vi "tutorialE11.vi"() -> ()   [LabVIEW 2017]
uses:
  Control 1.ctl
panel:
  in  "Delay (ms)":u32
  out "Count":dbl
  in  "# of Iterations":T1 scale=0.0..100.0
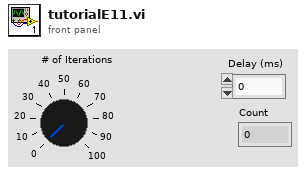
[diagram p1: front panel]
types:
  T1 = typedef "Control 1.ctl" = dbl
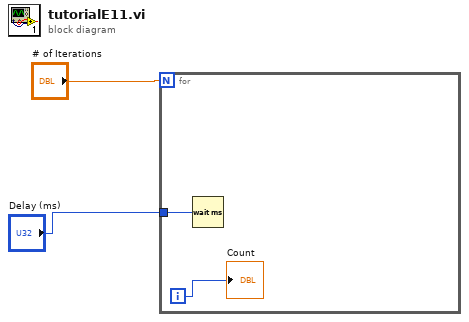
[diagram p0: block diagram]
diagram:
  n1 = for {
    N: "# of Iterations" -> [_]
    tunnel: "Delay (ms)" -> [w3]
    i -> [w4]
    n2 = Wait (ms)(milliseconds to wait=w3) -> ()  [unwired: 1 out]
    "Count" <- w4
  }
